vi "Demo_MicrophoneTest.vi"() -> ()   [LabVIEW 2018]
uses:
  PowerSupply4110/Type/SupplyConfig.ctl
  PowerSupply4110/Type/SupplyOutput.ctl
  Microfontest/Peiker_Stepped Sweep Settings.ctl
  <vilib>/addons/_NISVFA/_Shared subVIs/Controls/svc_DSA Channel Settings.ctl
  <vilib>/addons/_NISVFA/_Shared subVIs/Controls/svc_Channel Info.ctl
  <vilib>/addons/_NISVFA/_Shared subVIs/Controls/svc_Engineering Units Text Ring.ctl
  <vilib>/addons/_NISVFA/_Shared subVIs/Controls/svc_Weighting Filter Text Ring.ctl
  <instrlib>/niDCPower/nidcpower.llb/niDCPower Wait For Event - Event.ctl
panel:
  in  "Power on already?":bool
  out "Frequency list Input":T1(array[cluster])=[{"frequency [Hz]"=103.0, "amplitude [V]"=0.09342446715491094}] {"amplitude [V]" format="%.6f"; "frequency [Hz]" format="%.2f"}
  in  "Peiker_Stepped Sweep Settings":T2={"Input Settings"={"IEPE min time to settle [s]"=0.0, "Responce Channel Settings"={"DSA response channel settings"={"coupling"=10045, "enable IEPE excitation"=FALSE, "IEPE current [mA]"=4.0}, "response channel info"={"sensor sensitivity"=1000.0, "engineering units"=1, "dB reference"=1.0, "custom label"="EU", "weighting filter"=0, "pregain"=0.0}, "AI response settings"={"response channel"="SOUNDACQ/ai1", "max value [V]"=10.0, "min value [V]"=-10.0, "terminal configuration"=-1}}, "Stimulus Channel Settings"={"AI stimulus settings"={"stimulus channel"="SOUNDACQ/ai0", "max value [V]"=10.0, "min value [V]"=-10.0, "terminal configuration"=-1}, "DSA stimulus channel settings"={"coupling"=10045, "enable IEPE excitation"=FALSE, "IEPE current [mA]"=4.0}, "stimulus channel info"={"sensor sensitivity"=11.4, "engineering units"=2, "dB reference"=2e-05, "custom label"="EU", "weighting filter"=0, "pregain"=0.0}}}, "Output Settings"={"AO source settings"={"excitation channel"="SOUNDACQ/ao0", "max value [V]"=10.0, "min value [V]"=-10.0, "terminal configuration"=-1}}} {"Output Settings"."AO source settings"."terminal configuration" items=["Default"=-1, "RSE"=10083, "Differential"=10106, "Pseudodifferential"=12529]; "Output Settings"."AO source settings"."min value [V]" format="%0.2f"; "Output Settings"."AO source settings"."max value [V]" format="%0.2f"; "Input Settings"."Stimulus Channel Settings"."stimulus channel info"."pregain" format="%.2f"; "Input Settings"."Stimulus Channel Settings"."stimulus channel info"."weighting filter" items=["Linear", "A-weighting", "B-weighting", "C-weighting", "ITU-R 468-4", "Dolby", "CCITT", "C-message", "Wb", "Wc", "Wd", "We", "Wf", "Wh", "Wj", "Wk", "Wm", "AES17 20 kHz lowpass", "AES17 40 kHz lowpass", "AES17 20 kHz highpass", "AES17 40 kHz highpass"]; "Input Settings"."Stimulus Channel Settings"."stimulus channel info"."dB reference" format="%^.1e"; "Input Settings"."Stimulus Channel Settings"."stimulus channel info"."engineering units" items=["custom..."=0, "V"=1, "A"=21, "C"=30, "pC"=31, "s"=32, "-"=29, "Pa"=2, "N"=20, "g"=3, "m/s^2"=4, "m/s"=5, "m"=6, "mm/s"=12, "mm"=13, "micron/s"=14, "micron"=15, "in/s^2"=7, "in/s"=8, "in"=9, "mil/s"=10, "mil"=11, "rad/s^2"=16, "rad/s"=17, "rad"=18, "deg/s^2"=26, "deg/s"=27, "deg"=28, "RPM"=22, "cycle/s^2"=23, "Hz"=24, "cycle"=25, "strain"=19]; "Input Settings"."Stimulus Channel Settings"."stimulus channel info"."sensor sensitivity" format="%#_5f"; "Input Settings"."Stimulus Channel Settings"."DSA stimulus channel settings"."IEPE current [mA]" format="%.1f"; "Input Settings"."Stimulus Channel Settings"."DSA stimulus channel settings"."coupling" items=["AC"=10045, "DC"=10050, "GND"=10066]; "Input Settings"."Stimulus Channel Settings"."AI stimulus settings"."terminal configuration" items=["Default"=-1, "RSE"=10083, "NRSE"=10078, "Differential"=10106, "Pseudodifferential"=12529]; "Input Settings"."Stimulus Channel Settings"."AI stimulus settings"."min value [V]" format="%.2f"; "Input Settings"."Stimulus Channel Settings"."AI stimulus settings"."max value [V]" format="%.2f"; "Input Settings"."Responce Channel Settings"."AI response settings"."terminal configuration" items=["Default"=-1, "RSE"=10083, "NRSE"=10078, "Differential"=10106, "Pseudodifferential"=12529]; "Input Settings"."Responce Channel Settings"."AI response settings"."min value [V]" format="%.2f"; "Input Settings"."Responce Channel Settings"."AI response settings"."max value [V]" format="%.2f"; "Input Settings"."Responce Channel Settings"."response channel info"."pregain" format="%.2f"; "Input Settings"."Responce Channel Settings"."response channel info"."weighting filter" items=["Linear", "A-weighting", "B-weighting", "C-weighting", "ITU-R 468-4", "Dolby", "CCITT", "C-message", "Wb", "Wc", "Wd", "We", "Wf", "Wh", "Wj", "Wk", "Wm", "AES17 20 kHz lowpass", "AES17 40 kHz lowpass", "AES17 20 kHz highpass", "AES17 40 kHz highpass"]; "Input Settings"."Responce Channel Settings"."response channel info"."dB reference" format="%^.1e"; "Input Settings"."Responce Channel Settings"."response channel info"."engineering units" items=["custom..."=0, "V"=1, "A"=21, "C"=30, "pC"=31, "s"=32, "-"=29, "Pa"=2, "N"=20, "g"=3, "m/s^2"=4, "m/s"=5, "m"=6, "mm/s"=12, "mm"=13, "micron/s"=14, "micron"=15, "in/s^2"=7, "in/s"=8, "in"=9, "mil/s"=10, "mil"=11, "rad/s^2"=16, "rad/s"=17, "rad"=18, "deg/s^2"=26, "deg/s"=27, "deg"=28, "RPM"=22, "cycle/s^2"=23, "Hz"=24, "cycle"=25, "strain"=19]; "Input Settings"."Responce Channel Settings"."response channel info"."sensor sensitivity" format="%#_5f"; "Input Settings"."Responce Channel Settings"."DSA response channel settings"."IEPE current [mA]" format="%.1f"; "Input Settings"."Responce Channel Settings"."DSA response channel settings"."coupling" items=["AC"=10045, "DC"=10050, "GND"=10066]; "Input Settings"."IEPE min time to settle [s]" format="%.1f"}
  out "Init Frequency List":T1(array[cluster])
  in  "Tab Control":T7(tab)
  in  "AI - Response channel":tag="SOUNDACQ/ai1"
  in  "AO channel":tag="SOUNDACQ/ao0"
  in  "FrequencyListFilePath":path=path "D:/Valeo/Micriphone Test/Config/ME79_Limits.csv"
  in  "Response channel Setting":T4={"sensor sensitivity"=1000.0, "engineering units"=1, "dB reference"=1.0, "custom label"="EU", "weighting filter"=0, "pregain"=0.0} {"pregain" format="%.2f"; "weighting filter" items=["Linear", "A-weighting", "B-weighting", "C-weighting", "ITU-R 468-4", "Dolby", "CCITT", "C-message", "Wb", "Wc", "Wd", "We", "Wf", "Wh", "Wj", "Wk", "Wm", "AES17 20 kHz lowpass", "AES17 40 kHz lowpass", "AES17 20 kHz highpass", "AES17 40 kHz highpass"]; "dB reference" format="%^.1e"; "engineering units" items=["custom..."=0, "V"=1, "A"=21, "C"=30, "pC"=31, "s"=32, "-"=29, "Pa"=2, "N"=20, "g"=3, "m/s^2"=4, "m/s"=5, "m"=6, "mm/s"=12, "mm"=13, "micron/s"=14, "micron"=15, "in/s^2"=7, "in/s"=8, "in"=9, "mil/s"=10, "mil"=11, "rad/s^2"=16, "rad/s"=17, "rad"=18, "deg/s^2"=26, "deg/s"=27, "deg"=28, "RPM"=22, "cycle/s^2"=23, "Hz"=24, "cycle"=25, "strain"=19]; "sensor sensitivity" format="%#_5f"}
  in  "Stimulus channel Setting":T4={"sensor sensitivity"=1000.0, "engineering units"=1, "dB reference"=1.0, "custom label"="EU", "weighting filter"=0, "pregain"=0.0} {"pregain" format="%.2f"; "weighting filter" items=["Linear", "A-weighting", "B-weighting", "C-weighting", "ITU-R 468-4", "Dolby", "CCITT", "C-message", "Wb", "Wc", "Wd", "We", "Wf", "Wh", "Wj", "Wk", "Wm", "AES17 20 kHz lowpass", "AES17 40 kHz lowpass", "AES17 20 kHz highpass", "AES17 40 kHz highpass"]; "dB reference" format="%^.1e"; "engineering units" items=["custom..."=0, "V"=1, "A"=21, "C"=30, "pC"=31, "s"=32, "-"=29, "Pa"=2, "N"=20, "g"=3, "m/s^2"=4, "m/s"=5, "m"=6, "mm/s"=12, "mm"=13, "micron/s"=14, "micron"=15, "in/s^2"=7, "in/s"=8, "in"=9, "mil/s"=10, "mil"=11, "rad/s^2"=16, "rad/s"=17, "rad"=18, "deg/s^2"=26, "deg/s"=27, "deg"=28, "RPM"=22, "cycle/s^2"=23, "Hz"=24, "cycle"=25, "strain"=19]; "sensor sensitivity" format="%#_5f"}
  in  "AI - Stimulus channel":tag="SOUNDACQ/ai0"
  in  "Init Amplitude [V]":dbl=1.0
  in  "Power Supply":bool
  out "Supply Output":T8 {"Current mean" format="%.8f"; "Voltage mean" format="%.8f"; "Voltage min" format="%#_8g"; "Voltage max" format="%#_8g"; "Current min" format="%#_8g"; "Current max" format="%#_8g"}
  in  "PS settings":T9={"Channel Name"="0", "Source Delay (Sec)"=3.0, "Measurement:Sense"=1008, "voltage level"=5.0, "voltage level range"=6.0, "current limit"=0.02, "current limit range"=0.02, "resource name"="PSU"} {"current limit range" format="%_6p"; "current limit" format="%_6p"; "voltage level range" format="%_6p"; "voltage level" format="%_6p"; "Measurement:Sense" items=["Local"=1008, "Remote"=1009]; "Source Delay (Sec)" format="%_6p"}
  out "Voltage":waveform(dbl)(graph)
  out "Current":waveform(dbl)(graph)
  in  "RefMic Calibration":bool
  in  "Calibration settings":T10={"calibration value [dB SPL]"=94.0, "calibration frequency [Hz]"=1000.0}
  out "Calibrated sensor sensitivity [mV/Pa]":dbl=nan format="%.2g"
  in  "enable IEPE excitation (F)":bool
  out "power spectrum":cluster{"x0":dbl, "dx":dbl, "magnitude":dbl[]}(graph)
  in  "DAQmx physical channel":tag="SOUNDACQ/ai0"
  in  "Adjust Speaker":bool
  out "Corrected frequency list":T1(array[cluster])
  out "Magnitude":dbl[](array[numeric])
  in  "Set Level(dBSPL)":i32=94
  in  "integration time":T11={"integration time [s]"=0.03, "integration cycles"=5} {"integration cycles" min=2; "integration time [s]" format="%.2p"}
  in  "settling time":T12={"settle time [s]"=0.03, "settle cycles"=5} {"settle time [s]" format="%.2p"}
  in  "Test Frequency Response":bool
  out "Fundamental-Response":T13(graph)
  out "Response Level":cluster{"frequency":dbl[], "magnitude":dbl[]}(graph)
  out "Stimulus Level":cluster{"frequency":dbl[], "magnitude":dbl[]}(graph)
  in  "Frequency [Hz]":dbl=1000.0
  out "Sensitivity (dBSPL)":dbl
  out "Sensitivity Frequency (Hz)":dbl
  in  "THD Test":bool
  in  "Std_Deviation_Thresold":dbl=0.04 format="%#_13g"
  out "THD-Response":cluster{"frequency":dbl[], "THD":dbl[]}(graph)
  out "THD-Stimulus Level":cluster{"frequency":dbl[], "magnitude":dbl[]}(graph) caption="Stimulus Level"
  in  "THD Frequency":dbl=1000.0
  # "Power supply settings"
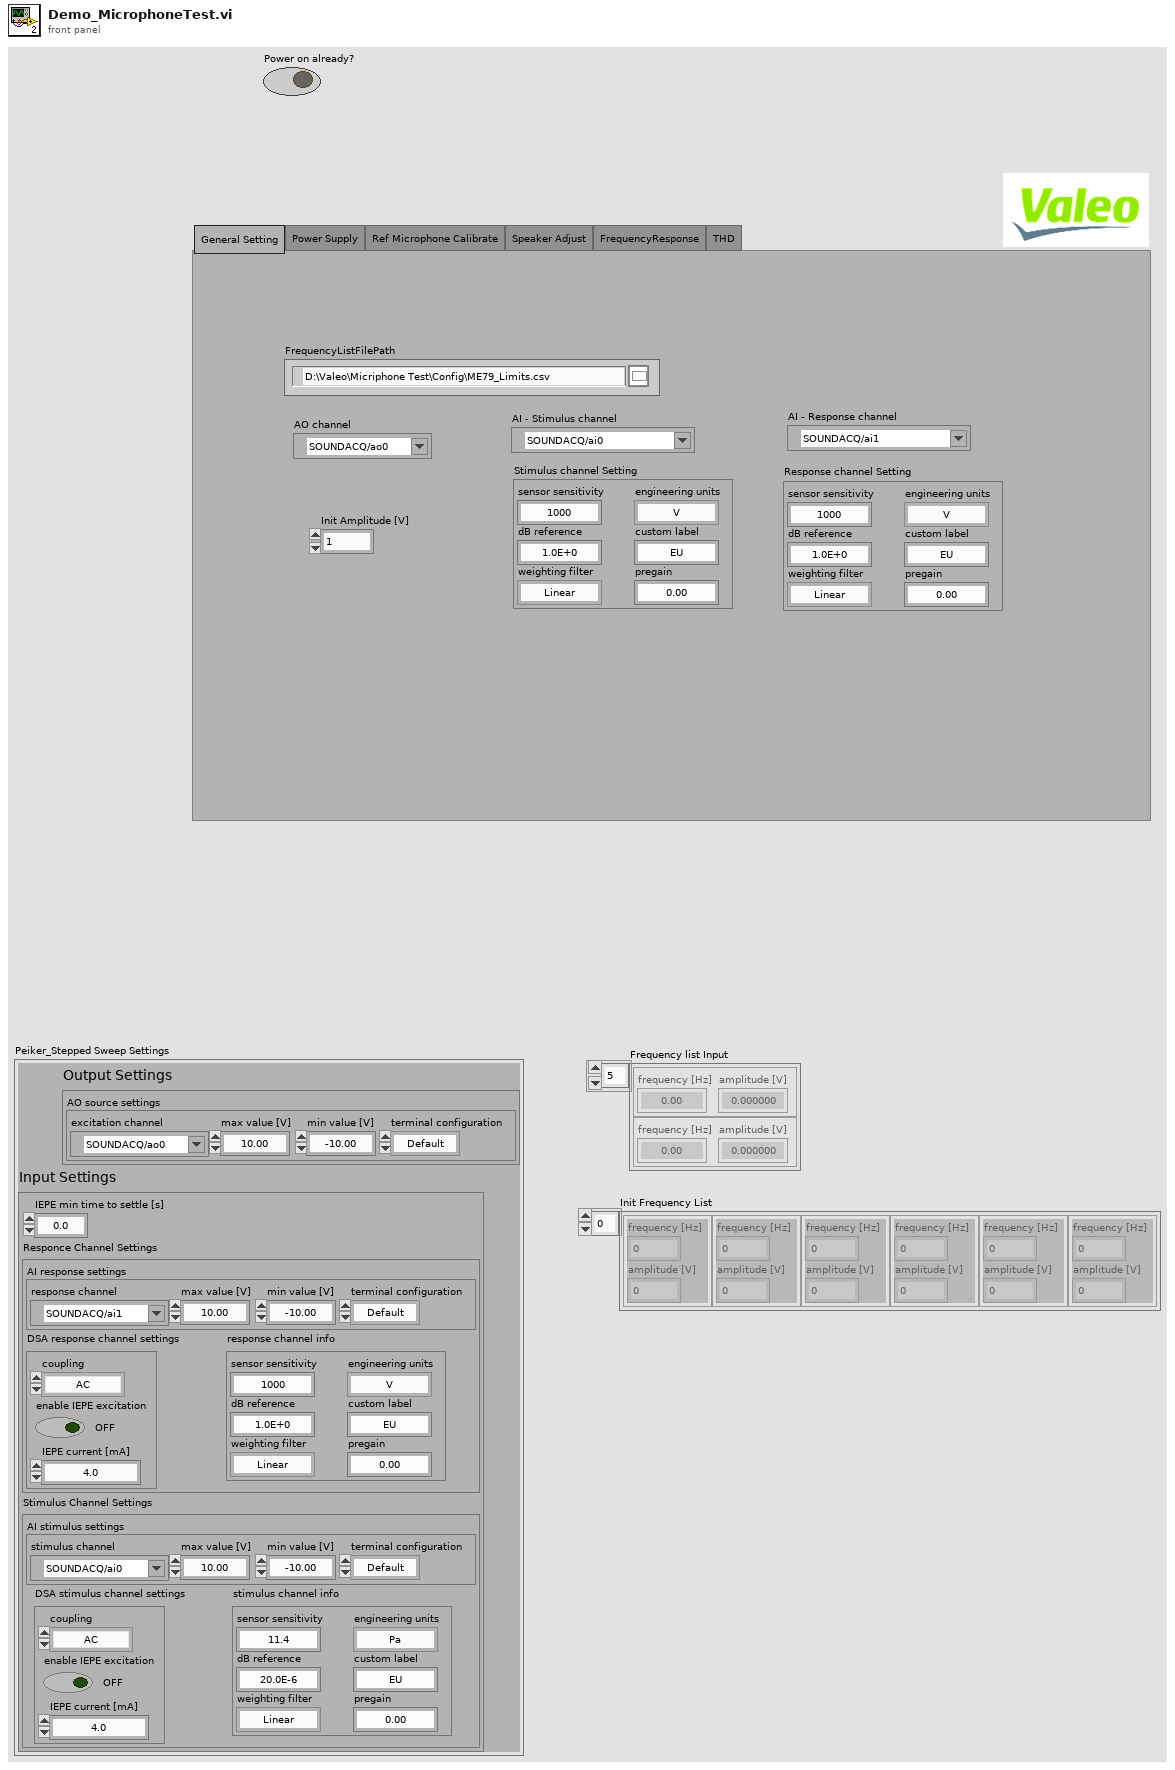
[diagram p1: front panel]
types:
  T1 = cluster{"frequency [Hz]":dbl, "amplitude [V]":dbl}[]
  T2 = typedef "Peiker_Stepped Sweep Settings.ctl" = cluster{"Input Settings":cluster{"IEPE min time to settle [s]":dbl, "Responce Channel Settings":cluster{"DSA response channel settings":T3, "response channel info":T4, "AI response settings":cluster{"response channel":tag, "max value [V]":dbl, "min value [V]":dbl, "terminal configuration":i32}}, "Stimulus Channel Settings":cluster{"AI stimulus settings":cluster{"stimulus channel":tag, "max value [V]":dbl, "min value [V]":dbl, "terminal configuration":i32}, "DSA stimulus channel settings":T3, "stimulus channel info":T4}}, "Output Settings":cluster{"AO source settings":cluster{"excitation channel":tag, "max value [V]":dbl, "min value [V]":dbl, "terminal configuration":i32}}}
  T3 = typedef "svc_DSA Channel Settings.ctl" = cluster{"coupling":i32, "enable IEPE excitation":bool, "IEPE current [mA]":dbl}
  T4 = typedef "svc_Channel Info.ctl" = cluster{"sensor sensitivity":dbl, "engineering units":T5, "dB reference":dbl, "custom label":string, "weighting filter":T6, "pregain":dbl}
  T5 = typedef "svc_Engineering Units Text Ring.ctl" = u16
  T6 = typedef "svc_Weighting Filter Text Ring.ctl" = u16
  T7 = enum32{"General Setting", "Power Supply", "Ref Microphone Calibrate", "Speaker Adjust", "FrequencyResponse", "THD"}
  T8 = typedef "SupplyOutput.ctl" = cluster{"Current max":dbl, "Current min":dbl, "Voltage max":dbl, "Voltage min":dbl, "Voltage mean":dbl, "Current mean":dbl}
  T9 = typedef "SupplyConfig.ctl" = cluster{"Channel Name":string, "Source Delay (Sec)":dbl, "Measurement:Sense":i32, "voltage level":dbl, "voltage level range":dbl, "current limit":dbl, "current limit range":dbl, "resource name":refnum<k15>}
  T10 = cluster{"calibration value [dB SPL]":dbl, "calibration frequency [Hz]":dbl}
  T11 = cluster{"integration time [s]":dbl, "integration cycles":i32}
  T12 = cluster{"settle time [s]":dbl, "settle cycles":i32}
  T13 = cluster{"frequency [Hz]":dbl[], "amplitude":dbl[]}
  T14 = cluster{"frequency [Hz]":dbl, "amplitude [V]":dbl}
  T15 = typedef "niDCPower Wait For Event - Event.ctl" = i32
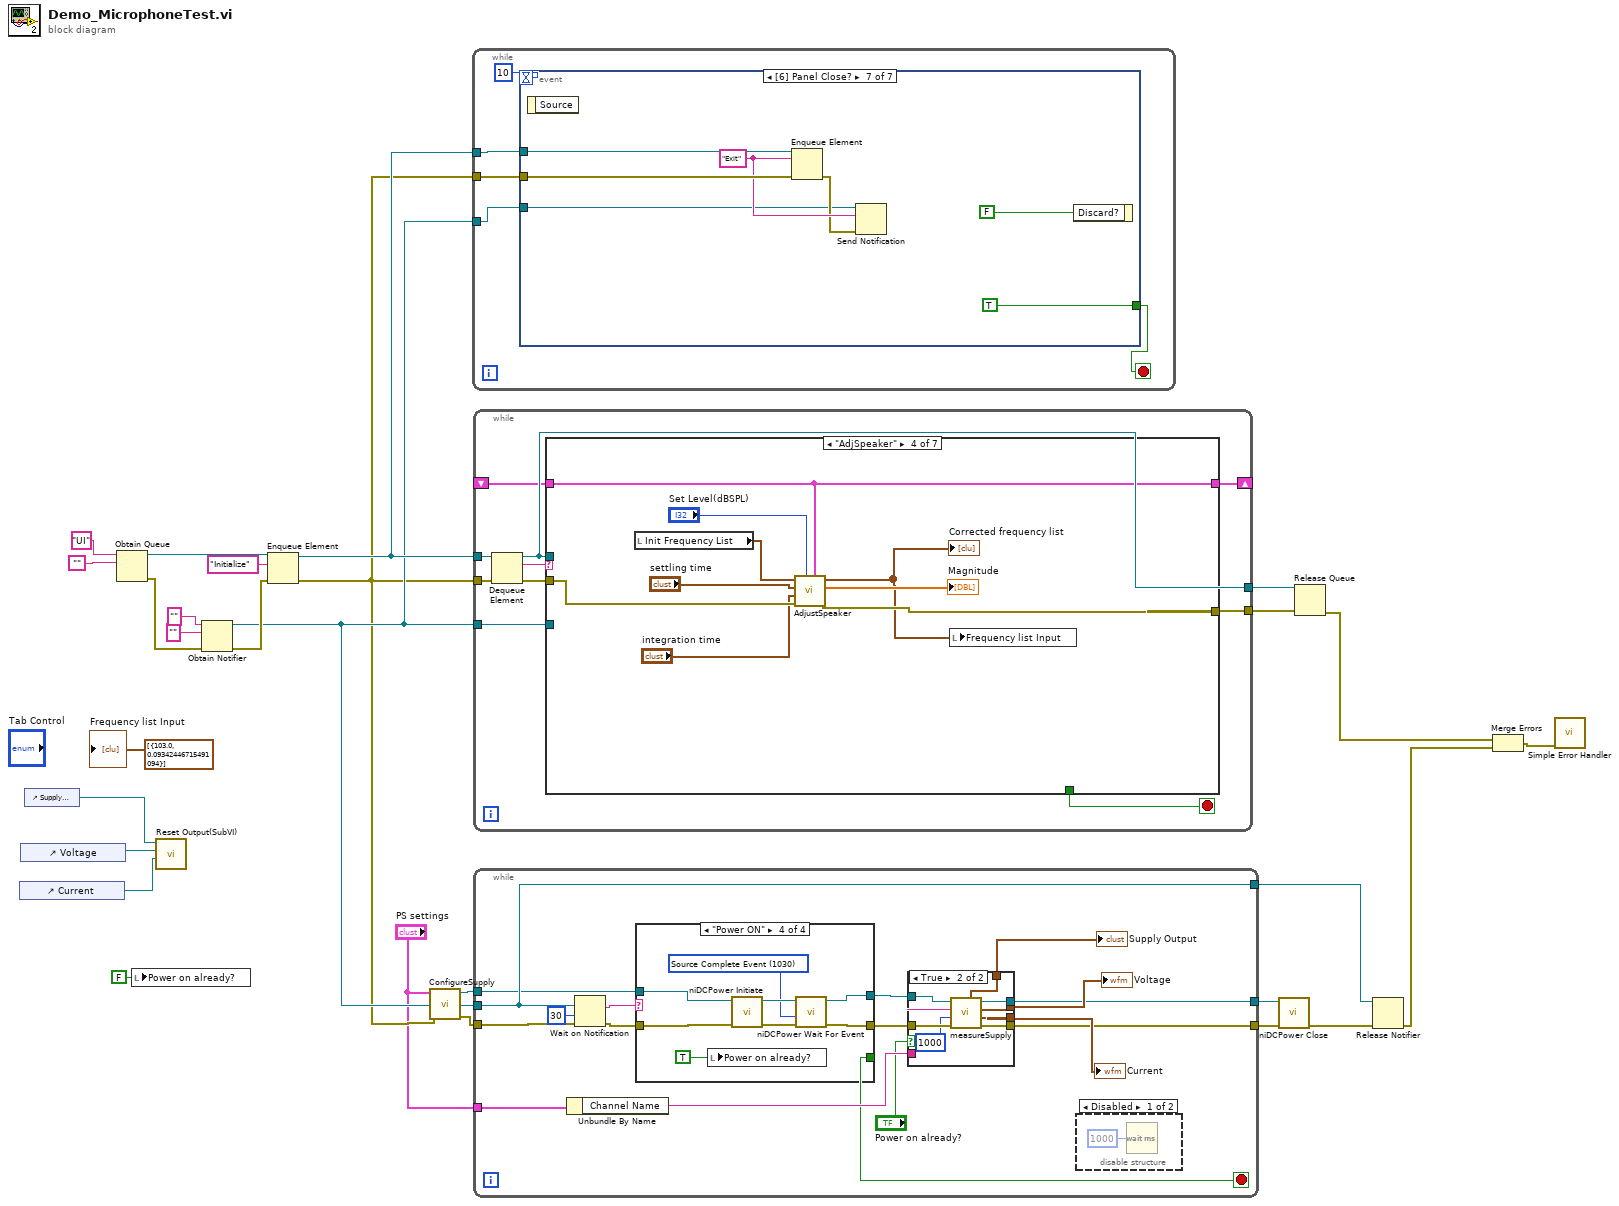
[diagram p0: block diagram]
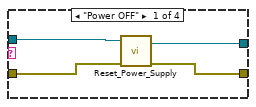
[diagram p4: hidden frame]
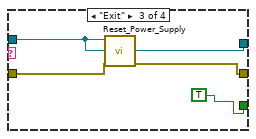
[diagram p6: hidden frame]
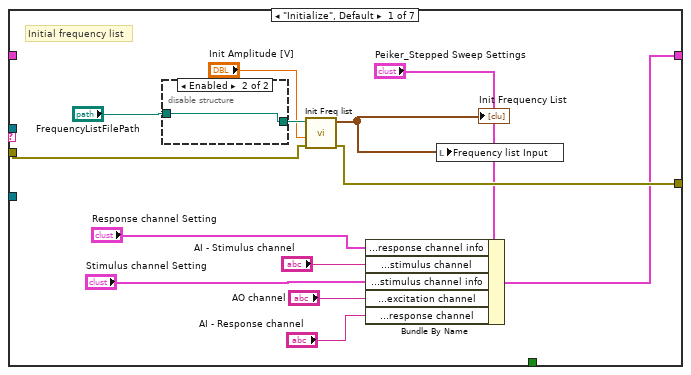
[diagram p7: hidden frame]
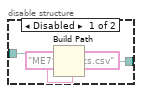
[diagram p8: hidden frame]
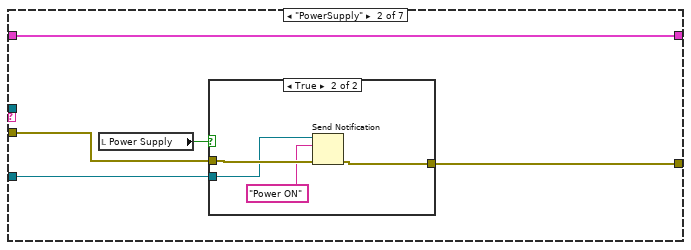
[diagram p9: hidden frame]
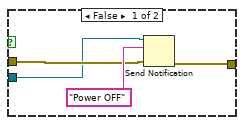
[diagram p10: hidden frame]
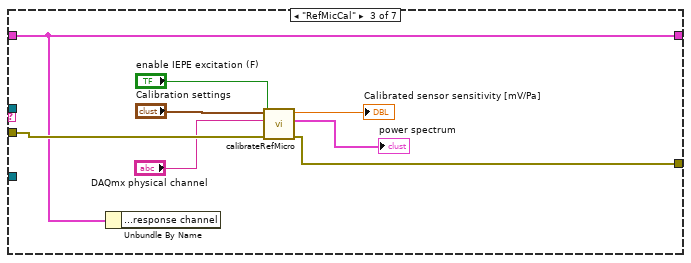
[diagram p11: hidden frame]
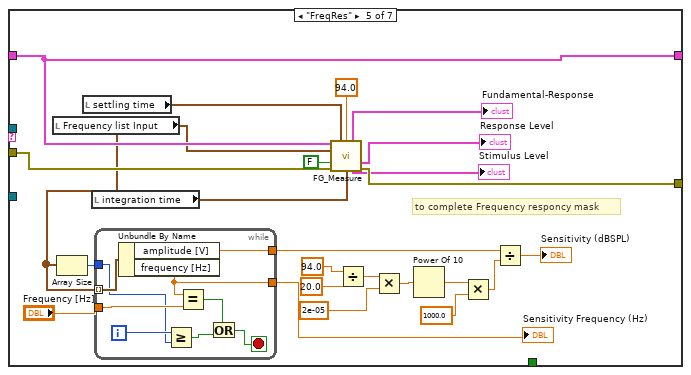
[diagram p12: hidden frame]
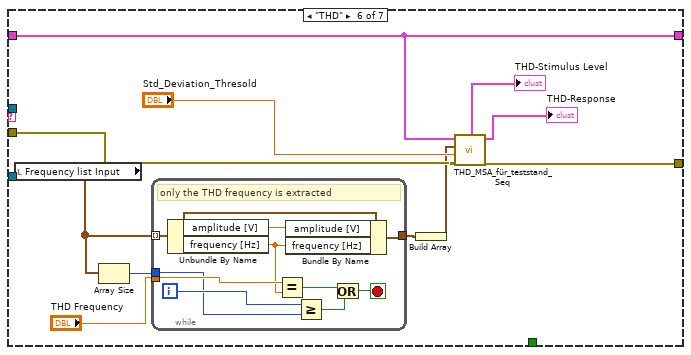
[diagram p13: hidden frame]
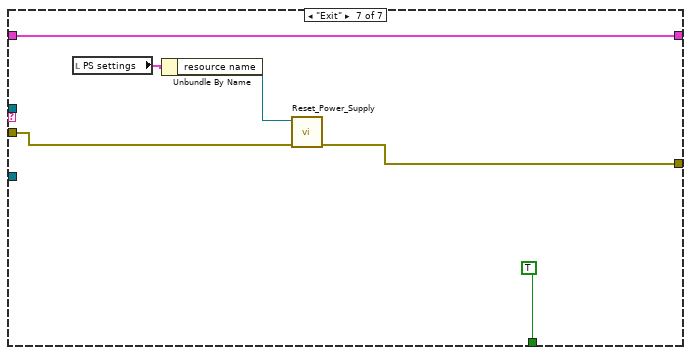
[diagram p14: hidden frame]
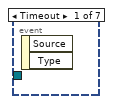
[diagram p15: hidden frame]
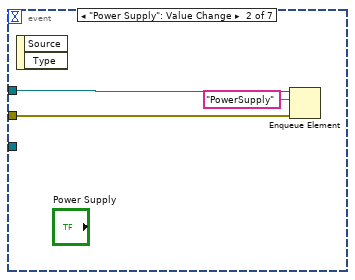
[diagram p16: hidden frame]
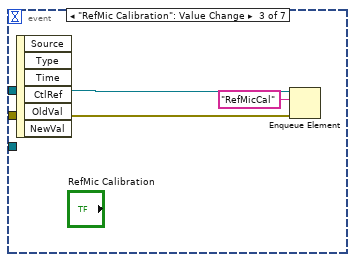
[diagram p17: hidden frame]
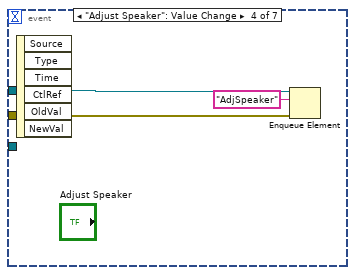
[diagram p18: hidden frame]
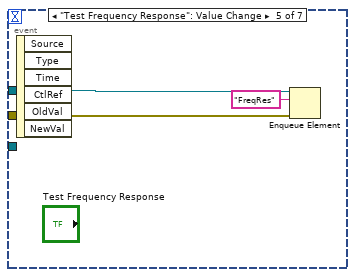
[diagram p19: hidden frame]
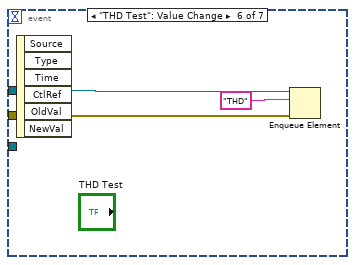
[diagram p20: hidden frame]
diagram:
  n1 = control-ref of="Current"() -> (w11:refnum<vi>)
  n2 = control-ref of="Voltage"() -> (w10:refnum<vi>)
  n3 = control-ref of="Supply Output"() -> (w9:refnum<vi>)
  n4 = Obtain Queue(name (unnamed)="UI", element data type="") -> (queue out=w28:refnum<queue>, error out=w18:errorcluster)  [unwired: 3 in, 1 out]
  n5 = local write "Power on already?"(FALSE ("Power on already?")) -> ()
  n6 = call "Reset Output(SubVI).vi"("WFGraph Refnum 2"=w11, "WFGraph Refnum"=w10, "Cluster in"=w9) -> ()  [unwired: 8 in, 1 out]
  n7 = Obtain Notifier(name (unnamed)="", notification data type="", error in (no error)=w18) -> (notifier out=w12:refnum<notifier>, error out=w15:errorcluster)  [unwired: 1 in, 1 out]
  n8 = Enqueue Element(queue=w28, element="Initialize", error in (no error)=w15) -> (queue out=w26:refnum<queue>, error out=w8:errorcluster)  [unwired: 1 in, 1 out]
  n9 = call "ConfigureSupply.vi"("error in (no error)"=w8, "Einstellungen"="PS settings") -> ("error out"=w7:errorcluster, "instrument handle out"=w6:refnum<k15>)  [unwired: 8 in]
  n10 = while {
    tunnel: w26 -> [w32]
    tunnel: w8 -> [w31]
    tunnel: w12 -> [w29]
    stop <- w30 stop-if-true
    n11 = event shown="[6] Panel Close?" {
      selector: _ -> [_ _ _ _ _ _ _]
      dyn-events: _ -> [_ _ _ _ _ _ _]
      timeout: 10 -> [_ _ _ _ _ _ _]
      tunnel: w32 -> [_ w36 w39 w42 w45 w48 w53]
      tunnel: w31 -> [_ w35 w38 w41 w44 w47 w52]
      tunnel: [_ _ _ _ _ _ TRUE] -> w30
      tunnel: w29 -> [_ _ _ _ _ _ w49]
      event Timeout {
        n12 = event-data() -> ()  [unwired: 1 in, 2 out]
      }
      event "Power Supply": Value Change {
        n13 = event-data() -> ()  [unwired: 1 in, 2 out]
        n14 = Enqueue Element(queue=w36, element="PowerSupply", error in (no error)=w35) -> ()  [unwired: 1 in, 3 out]
      }
      event "RefMic Calibration": Value Change {
        n15 = event-data() -> ()  [unwired: 1 in, 6 out]
        n16 = Enqueue Element(queue=w39, element="RefMicCal", error in (no error)=w38) -> ()  [unwired: 1 in, 3 out]
      }
      event "Adjust Speaker": Value Change {
        n17 = event-data() -> ()  [unwired: 1 in, 6 out]
        n18 = Enqueue Element(queue=w42, element="AdjSpeaker", error in (no error)=w41) -> ()  [unwired: 1 in, 3 out]
      }
      event "Test Frequency Response": Value Change {
        n19 = event-data() -> ()  [unwired: 1 in, 6 out]
        n20 = Enqueue Element(queue=w45, element="FreqRes", error in (no error)=w44) -> ()  [unwired: 1 in, 3 out]
      }
      event "THD Test": Value Change {
        n21 = event-data() -> ()  [unwired: 1 in, 6 out]
        n22 = Enqueue Element(queue=w48, element="THD", error in (no error)=w47) -> ()  [unwired: 1 in, 3 out]
      }
      event Panel Close? {
        w51 = "Exit" ("element")
        n23 = event-data() -> ()  [unwired: 1 in, 1 out]
        n24 = Enqueue Element(queue=w53, element=w51, error in (no error)=w52) -> (error out=w50:errorcluster)  [unwired: 1 in, 2 out]
        n25 = Send Notification(notification=w51, notifier=w49, error in (no error)=w50) -> ()  [unwired: 2 out]
        n26 = event-data("Discard?"=FALSE) -> ()  [unwired: 1 in, 1 out]
      }
    }
  }
  n27 = while {
    tunnel: w8 -> [w65]
    tunnel: w26 -> [w64]
    shift-right: [w58] -> _
    shift-left: _ -> [w57]
    tunnel: [w60] -> w25
    tunnel: [w59] -> w24
    tunnel: w12 -> [w56]
    stop <- w61 stop-if-true
    n28 = Dequeue Element(queue=w64, error in (no error)=w65) -> (queue out=w59:refnum<queue>, element=w63:string, error out=w62:errorcluster)  [unwired: 1 in, 1 out]
    n29 = case shown="\"AdjSpeaker\"" w63 {
      tunnel: w62 -> [w77 w86 w101 w112 w135 w154 w169]
      tunnel: w59 -> [_ _ _ _ _ _ _]
      tunnel: [_ _ _ _ _ _ TRUE] -> w61
      tunnel: [w76 w87 w100 w111 w134 w155 w168] -> w60
      tunnel: [w73 w85 w98 w104 w128 w151 w167] -> w58
      tunnel: w57 -> [_ w85 w98 w104 w128 w151 w167]
      tunnel: w56 -> [_ w83 _ _ _ _ _]
      frame "Initialize", Default {
        # "Initial frequency list"
        n30 = disable-structure shown="Enabled" {
          disable-tunnel: [w80 w82] -> w78
          disable-tunnel: "FrequencyListFilePath" -> [w79 w82]
          frame Disabled {
            n31 = Build Path(base path=w79, name or relative path="ME79_Limits.csv") -> (appended path=w80:path)
          }
          frame Enabled {
          }
        }
        n32 = call "Init Freq list.vi"("FrequencyListFile path"=w78, "Init Amplitude [V]"="Init Amplitude [V]", "error in (no error)"=w77) -> ("Frequency List"=w69:T1, "error out"=w76:errorcluster)  [unwired: 6 in]
        "Init Frequency List" <- w69
        n33 = Bundle By Name(cluster="Peiker_Stepped Sweep Settings", "Input Settings.Responce Channel Settings.response channel info"="Response channel Setting", "Input Settings.Stimulus Channel Settings.AI stimulus settings.stimulus channel"="AI - Stimulus channel", "Input Settings.Stimulus Channel Settings.stimulus channel info"="Stimulus channel Setting", "Output Settings.AO source settings.excitation channel"="AO channel", "Input Settings.Responce Channel Settings.AI response settings.response channel"="AI - Response channel") -> (w73:T2)
        n34 = local write "Frequency list Input"(w69) -> ()
      }
      frame "PowerSupply" {
        n35 = local read "Power Supply"() -> (w84:bool)
        n36 = case shown="True" w84 {
          tunnel: [w89 w94] -> w87
          tunnel: w86 -> [w90 w95]
          tunnel: w83 -> [w88 w93]
          frame False {
            n37 = Send Notification(notification="Power OFF", notifier=w88, error in (no error)=w90) -> (error out=w89:errorcluster)  [unwired: 1 out]
          }
          frame True {
            n38 = Send Notification(notification="Power ON", notifier=w93, error in (no error)=w95) -> (error out=w94:errorcluster)  [unwired: 1 out]
          }
        }
      }
      frame "RefMicCal" {
        n39 = Unbundle By Name(w98) -> ()  [unwired: 1 out]
        n40 = call "calibrateRefMicro.vi"("error in (no error)"=w101, "enable IEPE excitation (F)"="enable IEPE excitation (F)", "DAQmx physical channel"="DAQmx physical channel", "calibration settings"="Calibration settings") -> ("error out"=w100:errorcluster, "power spectrum"=→"power spectrum":cluster{"x0":dbl, "dx":dbl, "magnitude":dbl[]}, "calibrated sensor sensitivity [mV/Pa]"=→"Calibrated sensor sensitivity [mV/Pa]":dbl)  [unwired: 5 in]
      }
      frame "AdjSpeaker" {
        n41 = local read "Init Frequency List"() -> (w107:T1)
        n42 = call "AdjustSpeaker.vi"("Peiker_Stepped Sweep Settings"=w104, "Set level (dBSPL)"="Set Level(dBSPL)", "error in"=w112, "integration time"="integration time", "settling time"="settling time", "Frequency List"=w107) -> ("error out"=w111:errorcluster, "magnitude"=→"Magnitude":dbl[], "korrigierte Frequenzliste"=w108:T1)  [unwired: 3 in]
        "Corrected frequency list" <- w108
        n43 = local write "Frequency list Input"(w108) -> ()
      }
      frame "FreqRes" {
        # "to complete Frequency responcy mask"
        n44 = local read "Frequency list Input"() -> (w114:T1)
        n45 = Array Size(array=w114) -> (size(s)=w113:i32)
        n46 = local read "settling time"() -> (w130:T12)
        n47 = local read "integration time"() -> (w129:T11)
        n48 = while {
          tunnel: w114 -> [w145] mode=indexing
          tunnel: "Frequency [Hz]" -> [w144]
          tunnel: [w143] -> w125
          tunnel: [w142] -> w115
          tunnel: w113 -> [w138]
          i -> [w139]
          stop <- w141 stop-if-true
          n49 = Unbundle By Name(w145) -> ("amplitude [V]"=w143:dbl, "frequency [Hz]"=w142:dbl)
          n50 = Greater Or Equal?(x=w139, y=w138) -> (x >= y?=w137:bool)
          n51 = Equal?(x=w142, y=w144) -> (x = y?=w140:bool)
          n52 = Or(x=w140, y=w137) -> (x .or. y?=w141:bool)
        }
        "Sensitivity Frequency (Hz)" <- w115
        n53 = call "FG_Measure.vi"("Peiker_Stepped Sweep Settings"=w128, "settling time"=w130, "FrequencyList Output Level (dBSPL)"=94.0, "frequency list Input"=w114, "true=mehrfach Messen"=FALSE ("true = measure several times"), "error in (no error)"=w135, "integration time"=w129) -> ("Fundamental-Response"=→"Fundamental-Response":T13, "Response Level"=→"Response Level":cluster{"frequency":dbl[], "magnitude":dbl[]}, "Stimulus Level"=→"Stimulus Level":cluster{"frequency":dbl[], "magnitude":dbl[]}, "error out"=w134:errorcluster)  [unwired: 3 in, 2 out]
        n54 = Divide(x=94.0, y=20.0) -> (x/y=w122:dbl)
        n55 = Multiply(x=w122, y=2e-05) -> (x*y=w120:dbl)
        n56 = Power Of 10(x=w120) -> (10^x=w119:dbl)
        n57 = Multiply(x=w119, y=1000.0) -> (x*y=w117:dbl)
        n58 = Divide(x=w125, y=w117) -> (x/y=→"Sensitivity (dBSPL)":dbl)
      }
      frame "THD" {
        n59 = local read "Frequency list Input"() -> (w147:T1)
        n60 = Array Size(array=w147) -> (size(s)=w146:i32)
        n61 = while {
          tunnel: w147 -> [w162] mode=indexing
          tunnel: "THD Frequency" -> [w166]
          tunnel: [w163] -> w150
          tunnel: w146 -> [w157]
          i -> [w158]
          stop <- w159 stop-if-true
          # "only the THD frequency is extracted"
          n62 = Unbundle By Name(w162) -> ("amplitude [V]"=w164:dbl, "frequency [Hz]"=w165:dbl)
          n63 = Equal?(x=w166, y=w165) -> (x = y?=w160:bool)
          n64 = Bundle By Name(cluster=w162, "amplitude [V]"=w164, "frequency [Hz]"=w165) -> (w163:T14)
          n65 = Greater Or Equal?(x=w158, y=w157) -> (x >= y?=w161:bool)
          n66 = Or(x=w160, y=w161) -> (x .or. y?=w159:bool)
        }
        n67 = Build Array(w150) -> (w148:T1)
        n68 = call "THD_MSA_für_teststand_Seq.vi"("error in"=w154, "Std_Deviation_Thresold"="Std_Deviation_Thresold", "frequency list Input"=w148, "Peiker_Stepped Sweep Settings"=w151) -> ("error out"=w155:errorcluster, "Stimulus Level"=→"THD-Stimulus Level":cluster{"frequency":dbl[], "magnitude":dbl[]}, "THD-Response"=→"THD-Response":cluster{"frequency":dbl[], "THD":dbl[]})  [unwired: 5 in]
      }
      frame "Exit" {
        n69 = local read "PS settings"() -> (w171:T9)
        n70 = Unbundle By Name(w171) -> ("resource name"=w170:refnum<k15>)
        n71 = call "Reset_Power_Supply.vi"("error in (no error)"=w169, "resource name"=w170) -> ("error out"=w168:errorcluster)  [unwired: 9 in]
      }
    }
  }
  n72 = while {
    tunnel: w12 -> [w180]
    tunnel: w7 -> [w184]
    tunnel: [w180] -> w13
    tunnel: w6 -> [w177]
    tunnel: "PS settings" -> [w176]
    tunnel: [w175] -> w3
    tunnel: [w174] -> w2
    stop <- w179 stop-if-true
    n73 = Unbundle By Name(w176) -> ("Channel Name"=w183:string)
    n74 = Wait on Notification(notifier=w180, timeout in ms (-1)=30, error in (no error)=w184) -> (notification=w182:string, error out=w181:errorcluster)  [unwired: 1 in, 2 out]
    n75 = case shown="\"Power ON\"" w182 {
      tunnel: [w202 w206 w207 w216] -> w189
      tunnel: [w203 w205 w208 w215] -> w188
      tunnel: w181 -> [w204 w205 w209 w212]
      tunnel: [_ _ TRUE _] -> w179
      tunnel: w177 -> [w202 w206 w207 w213]
      frame "Power OFF" {
        n76 = call "Reset_Power_Supply.vi"("error in (no error)"=w204, "resource name"=w202) -> ("error out"=w203:errorcluster)  [unwired: 9 in]
      }
      frame Default {
      }
      frame "Exit" {
        n77 = call "Reset_Power_Supply.vi"("error in (no error)"=w209, "resource name"=w207) -> ("error out"=w208:errorcluster)  [unwired: 9 in]
      }
      frame "Power ON" {
        w214 = T15 1030 items=["Source Complete Event"=1030, "Measure Complete Event"=1031, "Sequence Iteration Complete Event"=1032, "Sequence Engine Done Event"=1033, "Pulse Complete Event"=1051, "Ready For Pulse Trigger Event"=1052] ("event")
        n78 = local write "Power on already?"(TRUE ("Power on already?")) -> ()
        n79 = call <instrlib>:"niDCPower Initiate.vi"("error in (no error)"=w212, "instrument handle"=w213) -> ("error out"=w217:errorcluster, "instrument handle out"=w218:refnum<k15>)  [unwired: 8 in]
        n80 = call <instrlib>:"niDCPower Wait For Event.vi"("error in (no error)"=w217, "event"=w214, "instrument handle"=w218) -> ("error out"=w215:errorcluster, "instrument handle out"=w216:refnum<k15>)  [unwired: 7 in]
      }
    }
    n81 = case shown="True" "Power on already?" {
      tunnel: w189 -> [w192 w201]
      tunnel: w188 -> [w191 w200]
      tunnel: [_ w199] -> w187
      tunnel: [_ w198] -> w186
      tunnel: [_ w197] -> w185
      tunnel: w183 -> [_ w196]
      tunnel: [w191 w195] -> w175
      tunnel: [w192 w194] -> w174
      frame False {
      }
      frame True {
        n82 = call "measureSupply.vi"("Supply instrument handle"=w201, "Supply Channel"=w196, "Messdauer/ms"=1000, "error in (no error)"=w200) -> ("Supply Output"=w197:T8, "Supply instrument handle"=w194:refnum<k15>, "Supply Voltage"=w198:waveform(dbl), "Supply Current"=w199:waveform(dbl), "error out"=w195:errorcluster)  [unwired: 2 in]
      }
    }
    "Voltage" <- w186
    "Current" <- w187
    "Supply Output" <- w185
    n83 = disable-structure shown="Disabled" {
      frame Disabled {
        n84 = Wait (ms)(milliseconds to wait=u32 1000) -> ()  [unwired: 1 out]
      }
      frame Enabled {
      }
    }
  }
  n85 = call <instrlib>:"niDCPower Close.vi"("error in (no error)"=w3, "instrument handle"=w2) -> ("error out"=w4:errorcluster)  [unwired: 9 in]
  n86 = Release Queue(queue=w24, error in (no error)=w25) -> (error out=w20:errorcluster)  [unwired: 1 in, 2 out]
  n87 = Release Notifier(notifier=w13, error in (no error)=w4) -> (error out=w14:errorcluster)  [unwired: 1 in, 2 out]
  n88 = Merge Errors(w20, w14) -> (w19:errorcluster)
  n89 = call <vilib>:"Simple Error Handler.vi"("error in (no error)"=w19) -> ()  [unwired: 4 in, 5 out]
  "Frequency list Input" <- T1 [{"frequency [Hz]"=103.0, "amplitude [V]"=0.09342446715491094}] ("frequency list Input")
